vi "5_2_inrangecomparison.vi"(10 "Map":T1(c390), 11 "Numeric":i64) -> (3 "element":i64)   [LabVIEW 2021, in "2023.lvlib"]
uses:
  2023.lvlib
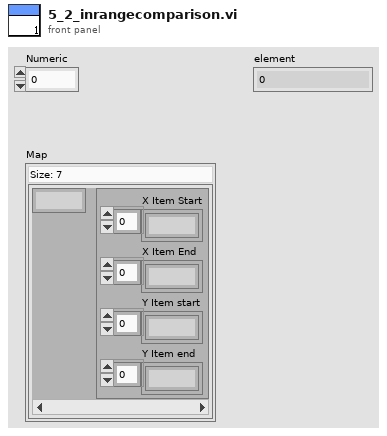
[diagram p1: front panel]
types:
  T1 = map{i32, cluster{"X Item Start":i64[], "X Item End":i64[], "Y Item start":i64[], "Y Item end":i64[]}}
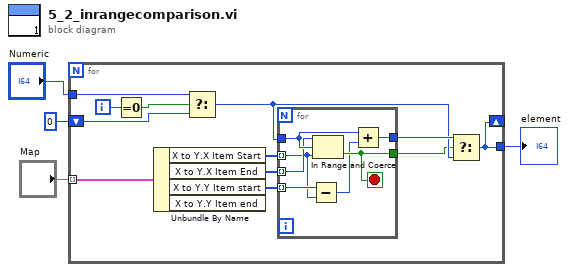
[diagram p0: block diagram]
diagram:
  n1 = for {
    tunnel: "Numeric" -> [w9]
    tunnel: "Map" -> [w16] mode=indexing
    shift-right: [w6] -> _
    shift-left: i64 0 ("element") -> [w8]
    tunnel: [w6] -> w4
    i -> [w11]
    n2 = Equal To 0?(x=w11) -> (x = 0?=w10:bool)
    n3 = Unbundle By Name(w16) -> ("X to Y.X Item Start"=w15:i64[], "X to Y.X Item End"=w14:i64[], "X to Y.Y Item start"=w13:i64[])  [unwired: 1 out]
    n4 = Select(t=w9, s=w10, f=w8) -> (s? t:f=w7:i64)
    n5 = for {
      tunnel: w15 -> [w17] mode=indexing
      tunnel: w14 -> [w19] mode=indexing
      tunnel: w7 -> [w22]
      tunnel: w13 -> [w20] mode=indexing
      tunnel: [w23] -> w5
      tunnel: [w21] -> w12
      stop <- w23 stop-if-true
      n6 = Subtract(x=w20, y=w17) -> (x-y=w18:i64)
      n7 = In Range and Coerce(upper limit=w19, x=w22, lower limit=w17) -> (In Range?=w23:bool)  [unwired: 1 out]
      n8 = Add(x=w22, y=w18) -> (x+y=w21:i64)
    }
    n9 = Select(t=w12, s=w5, f=w7) -> (s? t:f=w6:i64)
  }
  "element" <- w4
